vi "global_vars.vi"() -> ()   [LabVIEW 2011]
panel:
  out "Img Type":T1 items=["Grayscale (U8)", "Grayscale (I16)", "Grayscale (SGL)", "Complex (CSG)", "RGB (U32)", "HSL (U32)", "RGB (U64)", "Grayscale (U16)"]
  in  "UL_#Phase Shifts":i32
  in  "window size":cluster{"x Width(Px)":i32, "y height(Px)":i32}
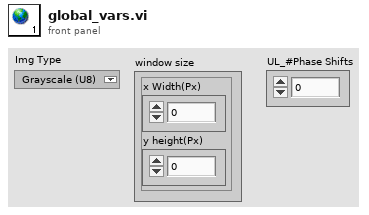
[diagram p1: front panel]
types:
  T1 = typedef "Image Type" = u32
diagram:
